vi "messages.vi"(6 "MaxLength (2000 Byte)":i32=2000, 9 "mode(Append)":enum16{"Append", "Clear", "Read"}(ring), 10 "Message":string) -> (1 "date string":string, 2 "Messages":string)   [LabVIEW 2019, in "Sending_larger_data.lvlib"]
uses:
  Sending_larger_data.lvlib
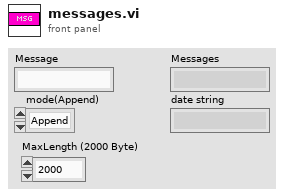
[diagram p1: front panel]
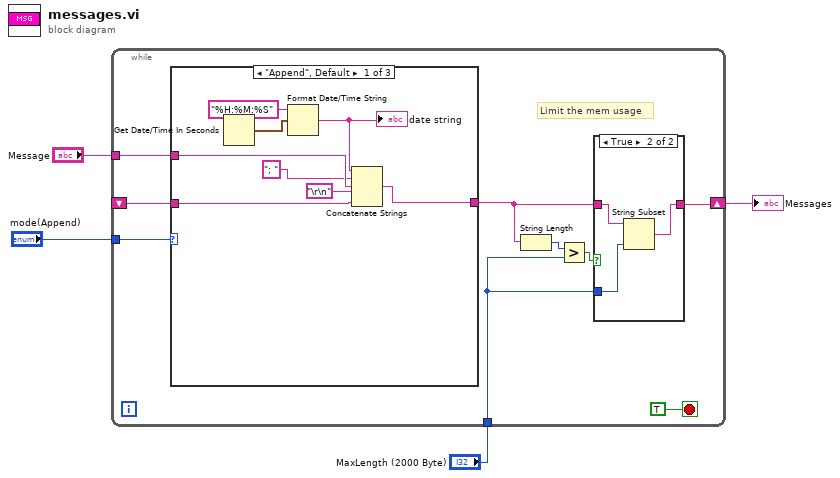
[diagram p0: block diagram]
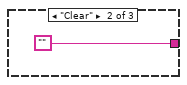
[diagram p3: hidden frame]
diagram:
  n1 = while {
    tunnel: "mode(Append)" -> [w12]
    shift-right: [w6] -> w2
    shift-left: _ -> [w11]
    tunnel: "Message" -> [w10]
    tunnel: "MaxLength (2000 Byte)" -> [w5]
    stop <- TRUE stop-if-true
    # "Limit the mem usage"
    n2 = case shown="\"Append\", Default" w12 {
      tunnel: w11 -> [w24 _ w27]
      tunnel: [w25 "" w27] -> w7
      tunnel: w10 -> [w22 _ _]
      frame "Append", Default {
        n3 = Get Date/Time In Seconds() -> (seconds since 1Jan1904=w21:timestamp)
        n4 = Format Date/Time String(time format string (%c)="%H:%M:%S", seconds (now)=w21) -> (date/time string=w19:string)  [unwired: 1 in]
        "date string" <- w19
        n5 = Concatenate Strings(w19, "; ", w22, "\r\n", w24) -> (w25:string)
      }
      frame "Clear" {
      }
      frame "Read" {
      }
    }
    n6 = String Length(string=w7) -> (length=w9:i32)
    n7 = Greater?(x=w9, y=w5) -> (0:w8:bool)
    n8 = case shown="True" w8 {
      tunnel: [w14 w16] -> w6
      tunnel: w7 -> [w14 w17]
      tunnel: w5 -> [_ w15]
      frame False {
      }
      frame True {
        n9 = String Subset(string=w17, length (rest)=w15) -> (substring=w16:string)  [unwired: 1 in]
      }
    }
  }
  "Messages" <- w2
